vi "Test UDP.vi"() -> ()   [LabVIEW 2015]
panel:
  in  "Boolean":bool
  in  "datagram":string
  in  "address":string
  in  "port or service name":u16
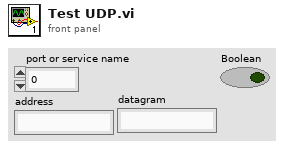
[diagram p1: front panel]
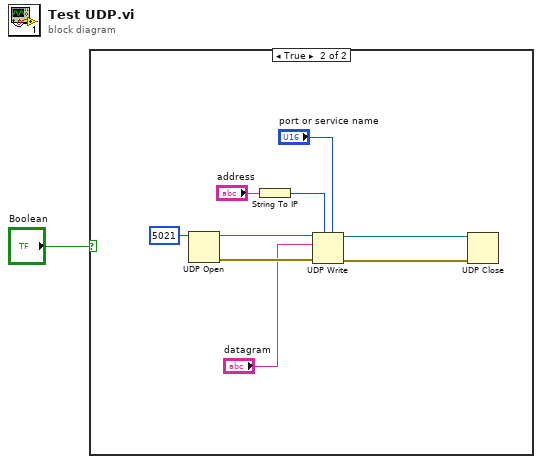
[diagram p0: block diagram]
diagram:
  n1 = case shown="True" "Boolean" {
    frame False {
    }
    frame True {
      n2 = UDP Open(11:u16 5021 ("port")) -> (port=w10:refnum<k16>, 0:w7:errorcluster)  [unwired: 4 in, 1 out]
      n3 = String To IP(1:"address") -> (0:w4:u32)
      n4 = UDP Write(address=w4, port or service name="port or service name", connection ID=w10, data in="datagram", 8:w7) -> (error out=w6:errorcluster, 3:w9:refnum<k16>)  [unwired: 1 in]
      n5 = UDP Close(connection ID=w9, 8:w6) -> ()  [unwired: 2 out]
    }
  }
